vi "PLC_OP20_Write.vi"(8 "error in (no error)":errorcluster, 10 "S7 Connection in":T1) -> (0 "error out":errorcluster, 3 "S7 Connection out":T1)   [LabVIEW 2017]
uses:
  <vilib>/DATA AHEAD/SP7/typedefs/S7 Connection.ctl
  <vilib>/DATA AHEAD/SP7/typedefs/PLC Type.ctl
  Global/DATA LOG.vi
  <vilib>/DATA AHEAD/SP7/functions/write/write Dint array.vi
  Global/Global 1.vi
  <vilib>/DATA AHEAD/SP7/functions/write/writeString.vi
  <vilib>/DATA AHEAD/SP7/SP7.lvlib
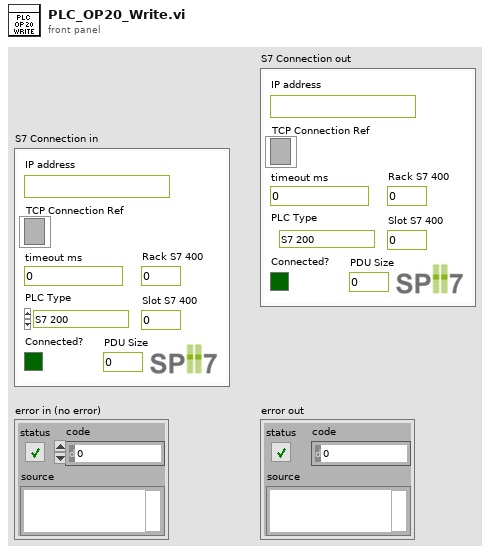
[diagram p1: front panel]
types:
  T1 = typedef "SP7.lvlib/S7 Connection.ctl" = cluster{"TCP Connection Ref":refnum<k5>, "IP address":string, "timeout ms":i32, "Connected?":bool, "PLC Type":T2, "Rack S7 400":u8, "Slot S7 400":u8, "PDU Size":u16, "connection semaphore":T3}
  T2 = typedef "SP7.lvlib/PLC Type.ctl" = enum16{"S7 200", "S7 300/400", "S7 1200", "S7 1500", "LOGO!8"}
  T3 = typedef "Semaphore RefNum" = refnum<k1>
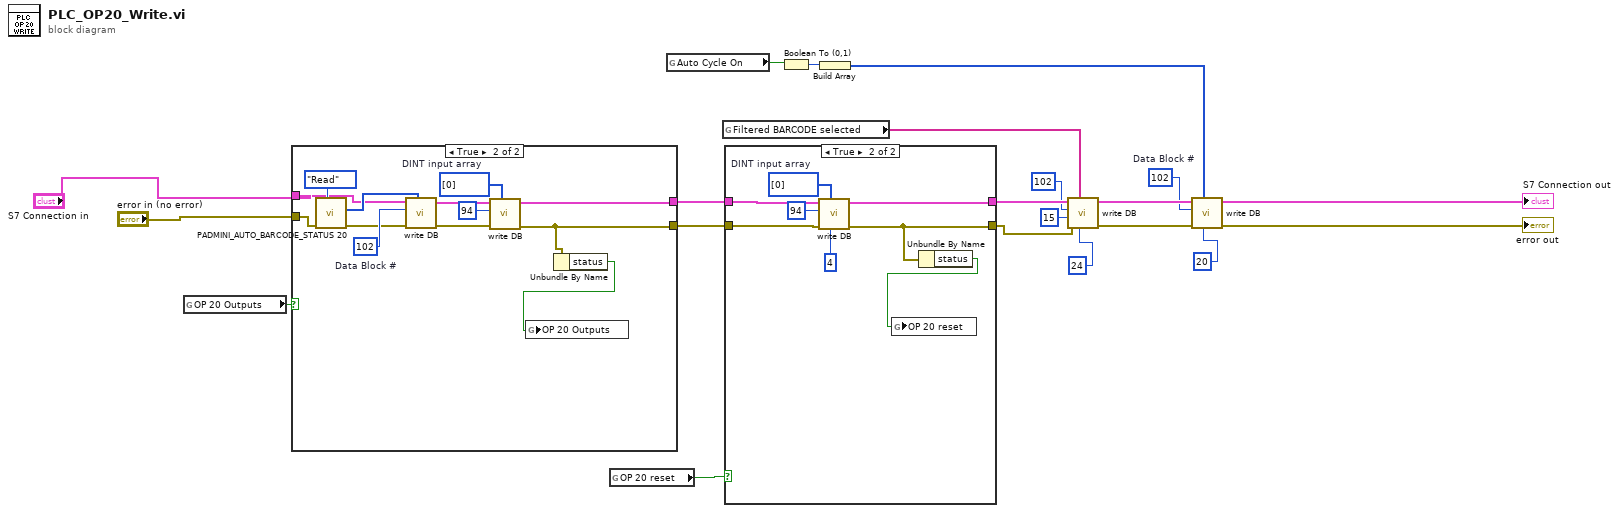
[diagram p0: block diagram]
diagram:
  w12 = u16 102  # Data Block #
  n1 = global read "DATA LOG.vi" "OP 20 Outputs"() -> (w5:bool)
  n2 = case shown="True" w5 {
    tunnel: [w23 w25] -> w18
    tunnel: [w22 w29] -> w19
    tunnel: "error in (no error)" -> [w23 w34]
    tunnel: "S7 Connection in" -> [w22 w31]
    frame False {
    }
    frame True {
      w30 = i32[] [0]  # DINT input array
      w36 = u16 102  # Data Block #
      n3 = call "PADMINI_AUTO_BARCODE_STATUS 20.vi"("Enum"=enum16{"Read", "Write"}."Read", "error in (no error)"=w34) -> ("error out"=w33:errorcluster, "O/P"=w32:i32[])  [unwired: 8 in]
      n4 = call-poly <vilib>:"write DB.vi"("DINT input array"=w32, "error in (no error)"=w33, "Data Block #"=w36, "S7 Connection in"=w31) -> ("error out"=w27:errorcluster, "S7 Connection out"=w28:T1)  [unwired: 4 in, 2 out]
      n5 = call-poly <vilib>:"write DB.vi"("DINT input array"=w30, "error in (no error)"=w27, "Data Block #"=u16 94, "S7 Connection in"=w28) -> ("error out"=w25:errorcluster, "S7 Connection out"=w29:T1)  [unwired: 4 in, 2 out]
      n6 = Unbundle By Name(w25) -> ("status"=w24:bool)
      n7 = global write "DATA LOG.vi" "OP 20 Outputs"(w24) -> ()
    }
  }
  n8 = global read "DATA LOG.vi" "OP 20 reset"() -> (w21:bool)
  n9 = global read "DATA LOG.vi" "Auto Cycle On"() -> (w3:bool)
  n10 = global read "Global 1.vi" "Filtered BARCODE selected"() -> (w4:string[])
  n11 = case shown="True" w21 {
    tunnel: [w37 w40] -> w17
    tunnel: [w38 w44] -> w20
    tunnel: w18 -> [w37 w42]
    tunnel: w19 -> [w38 w41]
    frame False {
    }
    frame True {
      w45 = i32[] [0]  # DINT input array
      n12 = call-poly <vilib>:"write DB.vi"("Item offset [byte]"=u32 4, "DINT input array"=w45, "error in (no error)"=w42, "Data Block #"=u16 94, "S7 Connection in"=w41) -> ("error out"=w40:errorcluster, "S7 Connection out"=w44:T1)  [unwired: 3 in, 2 out]
      n13 = Unbundle By Name(w40) -> ("status"=w39:bool)
      n14 = global write "DATA LOG.vi" "OP 20 reset"(w39) -> ()
    }
  }
  n15 = Boolean To (0,1)(Boolean=w3) -> (0, 1=w2:i16)
  n16 = Build Array(w2) -> (w1:i16[])
  n17 = call-poly <vilib>:"write DB.vi"("Item offset [byte]"=u32 24, "Input STRINGS"=w4, "error in (no error)"=w17, "String length reserved in DB (default=254)"=u16 15, "Data Block #"=u16 102, "S7 Connection in"=w20) -> ("error out"=w15:errorcluster, "S7 Connection out"=w13:T1)  [unwired: 2 in, 2 out]
  n18 = call-poly <vilib>:"write DB.vi"("Item offset [byte]"=u32 20, "DINT input array"=w1, "error in (no error)"=w15, "Data Block #"=w12, "S7 Connection in"=w13) -> ("error out"=→"error out":errorcluster, "S7 Connection out"=→"S7 Connection out":T1)  [unwired: 3 in, 2 out]
